vi "PaintFindedDisplac2.vi"(2 "error IN":errorcluster, 3 "Color of track":u32(colorbox)=16711680, 4 "Array of Points IN":dbl[](array[numeric]), 5 "Image IN":T1) -> (0 "error OUT":errorcluster, 1 "Image OUT":T1)   [LabVIEW 2013]
uses:
  <vilib>/vision/Image Controls.llb/IMAQ Image.ctl
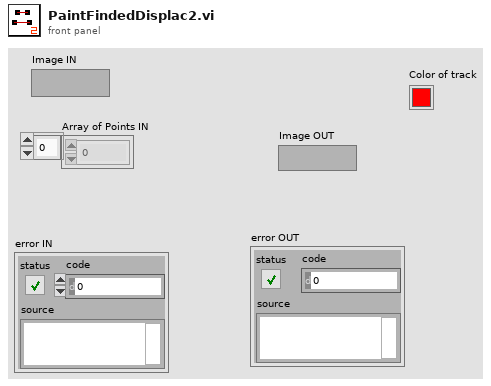
[diagram p1: front panel]
types:
  T1 = typedef "IMAQ Image.ctl" = refnum<image>
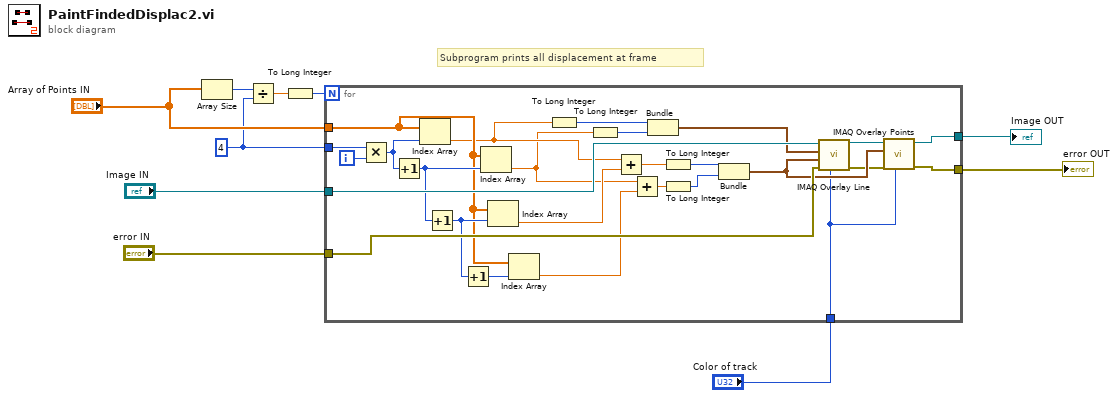
[diagram p0: block diagram]
diagram:
  w5 = 4 ("y")
  # "Subprogram prints all displacement at frame"
  n1 = Array Size(array="Array of Points IN") -> (size(s)=w10:i32)
  n2 = Divide(x=w10, y=w5) -> (x/y=w4:dbl)
  n3 = To Long Integer(number=w4) -> (32bit integer=w3:i32)
  n4 = for {
    N: w3 -> [_]
    tunnel: "Image IN" -> [w35]
    tunnel: "Array of Points IN" -> [w32]
    tunnel: "error IN" -> [w36]
    tunnel: [w26] -> w6
    tunnel: [w24] -> w1
    tunnel: w5 -> [w19]
    tunnel: "Color of track" -> [w11]
    i -> [w20]
    n5 = Multiply(x=w19, y=w20) -> (x*y=w17:i32)
    n6 = Increment(x=w17) -> (x+1=w34:i32)
    n7 = Index Array(array=w32, index=w17) -> (element=w15:dbl)
    n8 = Increment(x=w34) -> (x+1=w33:i32)
    n9 = Increment(x=w33) -> (x+1=w16:i32)
    n10 = Index Array(array=w32, index=w34) -> (element=w13:dbl)
    n11 = Index Array(array=w32, index=w33) -> (element=w30:dbl)
    n12 = Index Array(array=w32, index=w16) -> (element=w29:dbl)
    n13 = To Long Integer(number=w15) -> (32bit integer=w14:i32)
    n14 = To Long Integer(number=w13) -> (32bit integer=w12:i32)
    n15 = Add(x=w15, y=w30) -> (x+y=w21:dbl)
    n16 = Add(x=w13, y=w29) -> (x+y=w23:dbl)
    n17 = Bundle(w14, w12) -> (w31:cluster{i32, i32})  [unwired: 1 in]
    n18 = To Long Integer(number=w21) -> (32bit integer=w18:i32)
    n19 = To Long Integer(number=w23) -> (32bit integer=w22:i32)
    n20 = Bundle(w18, w22) -> (w27:cluster{i32, i32})  [unwired: 1 in]
    n21 = call "IMAQ Overlay Line"("Color"=w11, "error in (no error)"=w36, "End Point"=w27, "Start Point"=w31, "Image"=w35) -> ("error out"=w25:errorcluster, "Image Out"=w28:T1)  [unwired: 5 in]
    n22 = call "IMAQ Overlay Points"("Color"=w11, "error in (no error)"=w25, "Point"=w27, "Image"=w28) -> ("error out"=w24:errorcluster, "Image Out"=w26:T1)  [unwired: 6 in]
  }
  "Image OUT" <- w6
  "error OUT" <- w1
